vi "Chassis Info RTM.vi"(8 "error in (no error)":errorcluster, 11 "Node Ptr":u64 format="%.0x") -> (0 "error out":errorcluster)   [LabVIEW 2017, in "SLSC Switch System Explorer.lvlib"]
doc: "Demonstrates how to:\n- Discover SLSC devices\n- Reset SLSC devices\n- Rename SLSC devices\n- Add/remove SLSC chassis to/from the SLSC configuration file\n- Log in/out of an SLSC chassis, caching/deleting its login credentials\n- Update the firmware for an SLSC chassis\n- Open the web configuration page for an SLSC chassis"
uses:
  SLSC Switch System Explorer.lvlib
  SubVIs/ConfigurationStates.ctl
  <vilib>/NI Veristand/Custom Device API/Get Item Property (I32).vi
  <vilib>/nisyscfg/Close (System).vi
  <vilib>/SLSC/Initialize Session without Resources.vi
  <vilib>/SLSC/Initialize Session with Devices.vi
  <vilib>/SLSC/Close Session.vi
  <vilib>/Platform/browser.llb/Open URL in Default Browser (string).vi
  <vilib>/SLSC/SLSC.lvlib
  <resource>/objmgr/slsc.rc
  <vilib>/NI VeriStand/Custom Device API/Custom Device API.lvlib
  Scripting/VeriStand SLSC Scripting/VeriStand SLSC Scripting.lvlib
  <vilib>/nisyscfg/nisyscfg.lvlib
  <resource>/objmgr/nisysapi.rc
  <vilib>/Utility/SystemLogging/NI_SystemLogging.lvlib
panel:
  out "Name or IP":string
  out "Hostname":string
  in  "web config":bool
  in  "update firmware":bool
  out "device properties":string[][](table)
  in  "refresh":bool
  in  "logout":bool
  in  "login":bool
  in  "rename":bool
  in  "reset":bool
  in  "stop":bool
  in  "remove":bool
  in  "add":bool
  in  "devices":string(tree)="jasonSlsc-5"
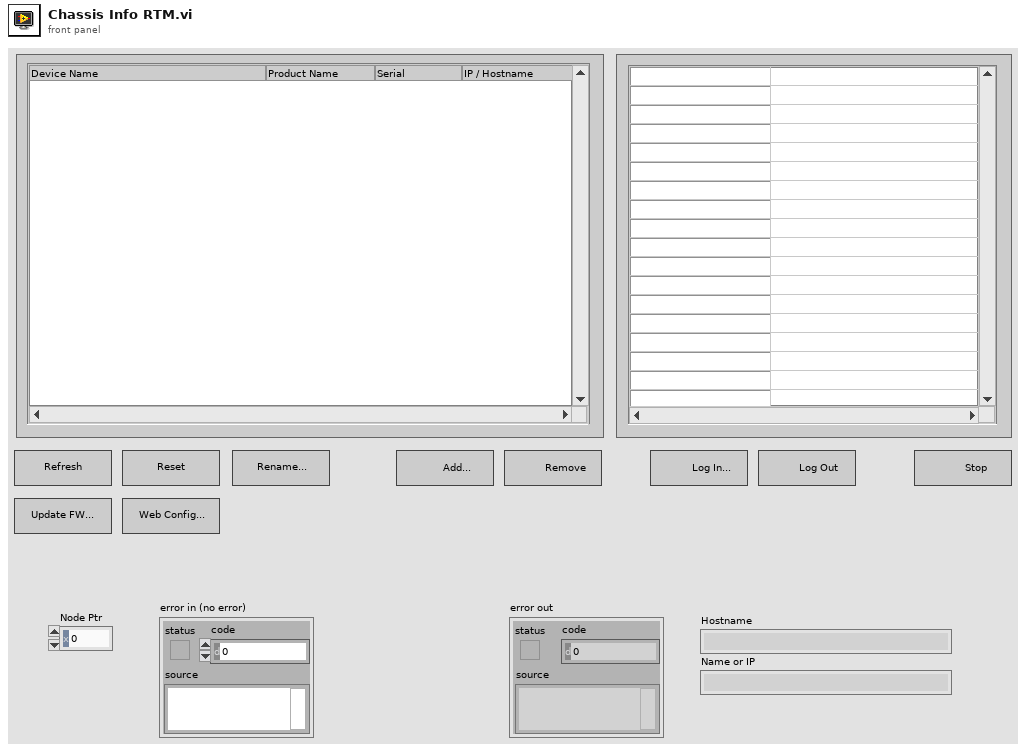
[diagram p1: front panel]
types:
  T1 = typedef "ConfigurationStates.ctl" = enum16{"Add", "Remove", "Rename", "Reset", "Login", "Logout", "Stop", "Refresh", "Update Firmware", "Web Config"}
  T2 = typedef "Custom Device API.lvlib/Custom Device Item Ref.ctl" = u64
  T3 = enum8{"Enabled", "Disabled", "Disabled and Grayed Out"}
  T4 = typedef "VeriStand SLSC Scripting.lvlib/SLSC Chassis ID.ctl" = cluster{"Name or IP":string, "ChassisIDType":i32, "chassisType":i32}
  T5 = enum32{"Invalid", "Standard", "Closed", "Hidden", "Minimized", "Maximized"}
  T6 = cluster{"hostname":string, "username":string, "password":string}
  T7 = cluster{"username":string, "password":string, "save credentials to disk":bool}
  T8 = cluster{"firmware path":path, "username":string, "password":string}
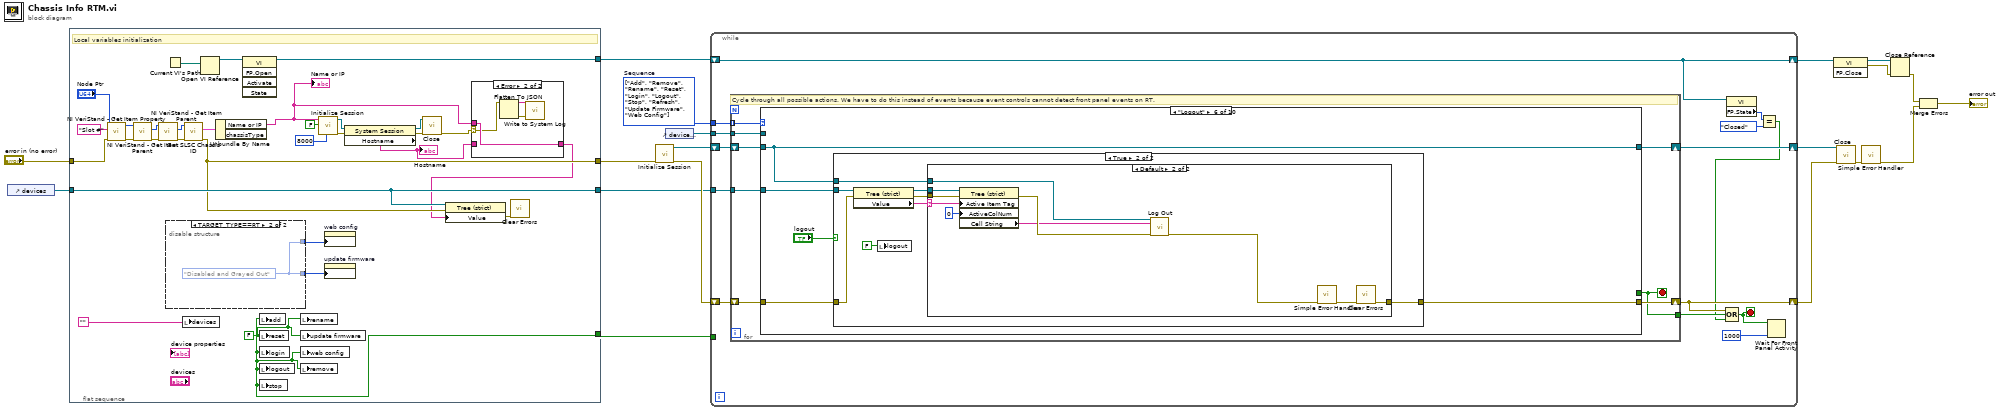
[diagram p0: block diagram]
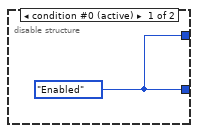
[diagram p3: hidden frame]
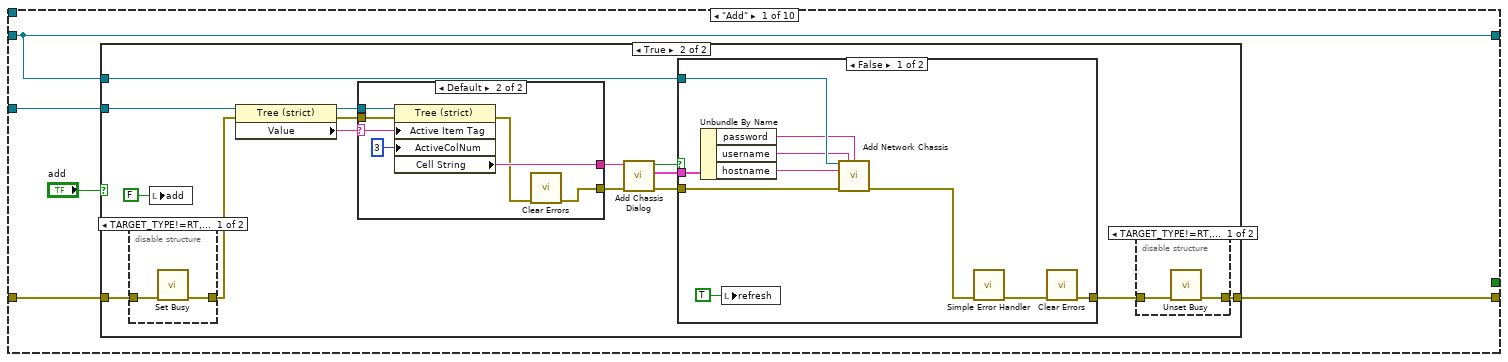
[diagram p4: hidden frame]
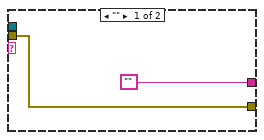
[diagram p6: hidden frame]
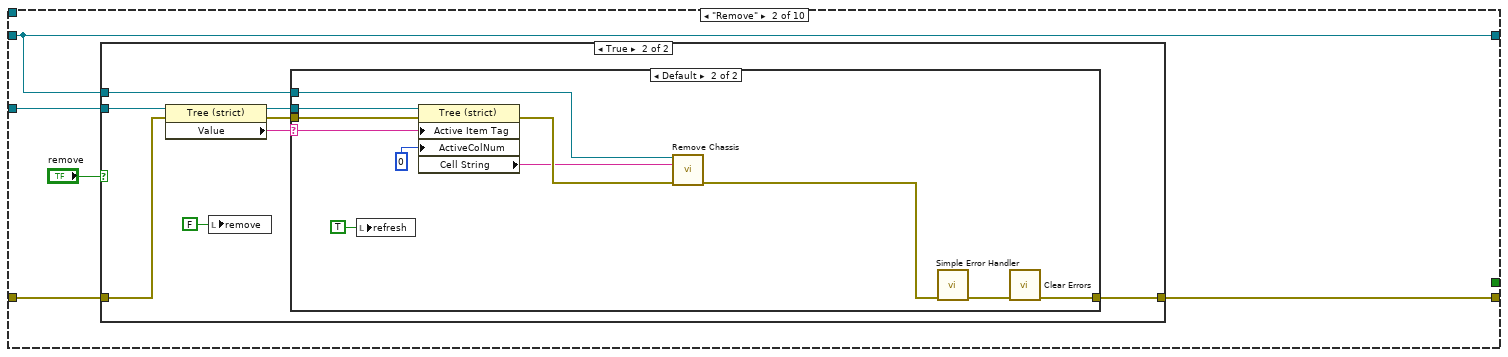
[diagram p10: hidden frame]
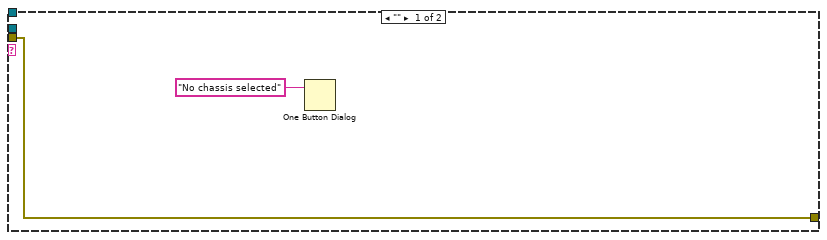
[diagram p12: hidden frame]
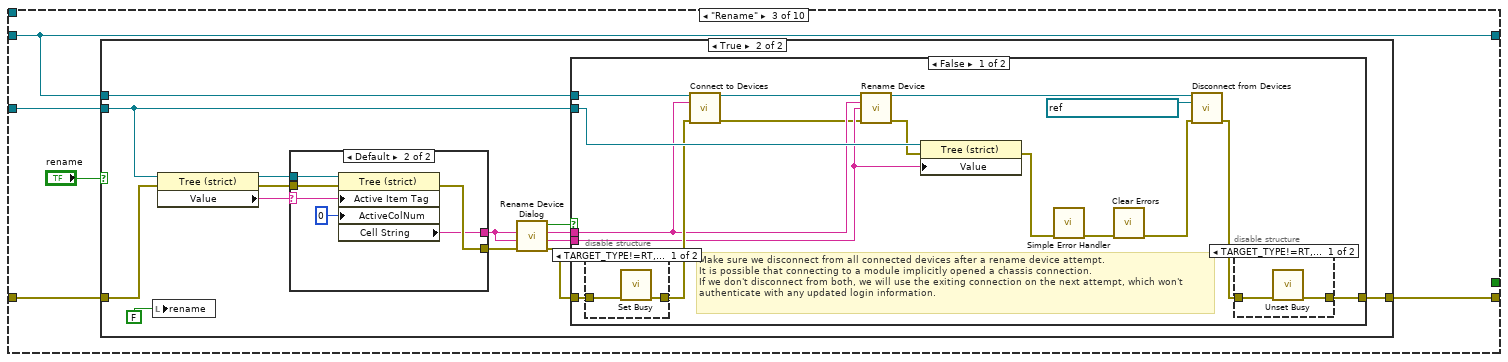
[diagram p13: hidden frame]
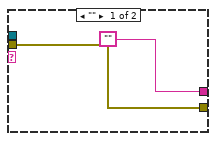
[diagram p15: hidden frame]
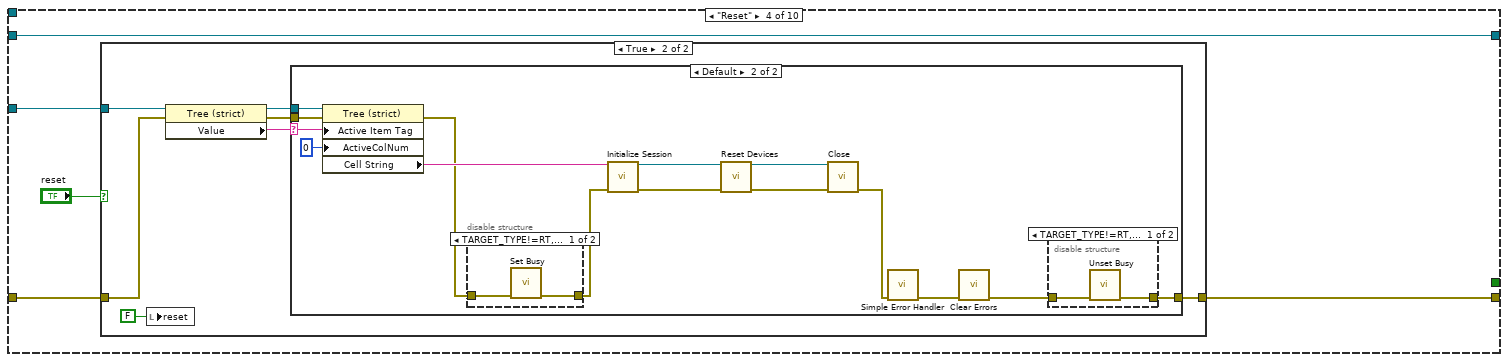
[diagram p19: hidden frame]
diagram:
  w15 = T1[] [enum."Add", enum."Remove", enum."Rename", enum."Reset", enum."Login", enum."Logout", enum."Stop", enum."Refresh", enum."Update Firmware", enum."Web Config"] items=["Add", "Remove", "Rename", "Reset", "Login", "Logout", "Stop", "Refresh", "Update Firmware", "Web Config"]  # Sequence
  n1 = control-ref of="devices"() -> (w6:refnum<vi>)
  n2 = flat-sequence {
    tunnel: [w49] -> w14
    tunnel: "error in (no error)" -> [w35]
    tunnel: [w24] -> w10
    tunnel: [w43] -> w9
    tunnel: [w34] -> w7
    tunnel: w6 -> [w34]
    frame #0 {
      w49 = FALSE
      # "Local variables initialization"
      n3 = call-poly <vilib>:"NI VeriStand - Get Item Property.vi"("error in (no error)"=w35, "Property Name"="Slot #", "Item Ref in"="Node Ptr") -> ("error out"=w39:errorcluster, "Item Ref out"=w38:T2)  [unwired: 5 in, 2 out]
      n4 = call <vilib>:"NI VeriStand - Get Item Parent.vi"("error in (no error)"=w39, "Item Ref in"=w38) -> ("error out"=w40:errorcluster, "Parent Ref"=w37:T2)  [unwired: 6 in, 2 out]
      n5 = call <vilib>:"NI VeriStand - Get Item Parent.vi"("error in (no error)"=w40, "Item Ref in"=w37) -> ("error out"=w41:errorcluster, "Parent Ref"=w32:T2)  [unwired: 6 in, 2 out]
      n6 = disable-structure shown="TARGET_TYPE==RT" {
        disable-tunnel: [w55 w56] -> w48
        disable-tunnel: [w55 w56] -> w46
        frame condition #0 (active) {
          w55 = T3."Enabled" ("Disabled")
        }
        frame condition #1 {
          w56 = T3."Disabled and Grayed Out" ("Disabled")
        }
      }
      n7 = Current VI's Path() -> (path=w45:path)
      n8 = local write "devices"("") -> ()
      n9 = call "Get SLSC Chassis ID.vi"("error in (no error)"=w41, "SLSC Chassis Ref in"=w32) -> ("error out"=w24:errorcluster, "SLSC Chassis ID"=w27:T4)  [unwired: 7 in, 1 out]
      n10 = Open VI Reference(vi path=w45) -> (vi reference=w44:refnum<vi>)  [unwired: 5 in, 1 out]
      n11 = Unbundle By Name(w27) -> ("Name or IP"=w20:string)  [unwired: 1 out]
      "Name or IP" <- w20
      n12 = invoke class="VI" method="FP.Open"(reference=w44) -> (reference out=w43:refnum<vi>)  [unwired: 4 in, 4 out]
      n13 = local write "add"(w49) -> ()
      n14 = local write "reset"(w49) -> ()
      n15 = local write "login"(w49) -> ()
      n16 = local write "logout"(w49) -> ()
      n17 = local write "stop"(w49) -> ()
      n18 = local write "rename"(w49) -> ()
      n19 = local write "update firmware"(w49) -> ()
      n20 = local write "web config"(w49) -> ()
      n21 = local write "remove"(w49) -> ()
      n22 = call <vilib>:"Initialize Session.vi"("Connect Timeout (4000 ms)"=u32 8000, "Force Property Refresh (T)"=FALSE, "Target (localhost)"=w20) -> ("error out"=w30:errorcluster, "Session out"=w31:refnum<k21>)  [unwired: 7 in]
      n23 = property on="web config" class="Bool (strict)"("DisabledEnum"=w46) -> ()  [unwired: 2 in, 2 out]
      n24 = property on="update firmware" class="Bool (strict)"("DisabledEnum"=w48) -> ()  [unwired: 2 in, 2 out]
      n25 = property class="System Session"(reference=w31, error in=w30) -> (reference out=w28:refnum<k21>, error out=w26:errorcluster, "Hostname"=w22:string)
      "Hostname" <- w22
      n26 = call-poly <vilib>:"Close.vi"("error in (no error)"=w26, "Session in"=w28) -> ("error out"=w23:errorcluster)  [unwired: 9 in]
      n27 = case shown="Error" w23 {
        selector: w23 -> [_ w51]
        tunnel: w22 -> [w50 _]
        tunnel: [w50 w54] -> w21
        tunnel: w20 -> [_ w54]
        frame No Error {
        }
        frame Error {
          n28 = Flatten To JSON(anything=w51) -> (JSON string=w52:string, 11:w53:errorcluster)  [unwired: 2 in]
          n29 = call <vilib>:"Write to System Log.vi"("error in (no error)"=w53, "message"=w52) -> ()  [unwired: 9 in, 1 out]
        }
      }
      n30 = property class="Tree (strict)"(reference=w34, error in=w24, "Value"=w21) -> (error out=w33:errorcluster)  [unwired: 1 out]
      n31 = call <vilib>:"Clear Errors.vi"("error in (no error)"=w33) -> ()  [unwired: 5 in, 2 out]
    }
  }
  n32 = call-poly <vilib>:"Initialize Session.vi"("error in (no error)"=w10) -> ("session out"=w16:refnum<k21>, "error out"=w19:errorcluster)  [unwired: 13 in]
  n33 = control-ref of="device properties"() -> (w12:refnum<vi>)
  n34 = while {
    shift-right: [w68] -> w18
    shift-left: w19 -> [w70]
    tunnel: w7 -> [w61]
    tunnel: w15 -> [w66]
    tunnel: w14 -> [_]
    shift-right: [w65] -> w13
    shift-left: w16 -> [w69]
    tunnel: w12 -> [w62]
    shift-right: [w60] -> w8
    shift-left: w9 -> [w60]
    stop <- w63 stop-if-true
    n35 = for {
      tunnel: [w73] -> w67
      tunnel: w61 -> [w75]
      shift-right: [w76] -> w68
      shift-left: w70 -> [w78]
      tunnel: w66 -> [w74] mode=indexing
      shift-right: [w72] -> w65
      shift-left: w69 -> [w77]
      tunnel: w62 -> [w71]
      stop <- w73 stop-if-true
      # "Cycle through all possible actions. We have to do this instead of events because event controls cannot detect front panel events on RT."
      n36 = case shown="\"Logout\"" w74 {
        tunnel: w78 -> [w82 w128 w156 w206 w243 w288 w313 w342 w413 w470]
        tunnel: w77 -> [w80 w126 w153 w204 w240 w285 w311 w334 w411 w472]
        tunnel: [w81 w127 w155 w205 w241 w286 w313 w319 w412 w469] -> w76
        tunnel: [_ _ _ _ _ _ "stop" _ _ _] -> w73
        tunnel: w75 -> [w79 w129 w157 w207 w242 w287 _ w336 w414 w473]
        tunnel: [w80 w126 w153 w204 w240 w285 w311 w339 w410 w471] -> w72
        tunnel: w71 -> [_ _ _ _ _ _ _ w337 _ _]
        frame "Add" {
          n37 = case shown="True" "add" {
            tunnel: w82 -> [w84 w98]
            tunnel: w80 -> [_ w97]
            tunnel: [w84 w96] -> w81
            tunnel: w79 -> [_ w85]
            frame False {
            }
            frame True {
              n38 = disable-structure shown="TARGET_TYPE!=RT, Default" {
                disable-tunnel: w98 -> [w113 w114]
                disable-tunnel: [w112 w114] -> w86
                frame condition #0 (active) {
                  n39 = call <vilib>:"Set Busy.vi"("error in (no error)"=w113) -> ("error out"=w112:errorcluster)  [unwired: 9 in, 1 out]
                }
                frame condition #1 {
                }
              }
              n40 = local write "add"(FALSE ("stop")) -> ()
              n41 = property class="Tree (strict)"(reference=w85, error in=w86) -> (reference out=w90:refnum<vi>, error out=w89:errorcluster, "Value"=w91:string)
              n42 = case shown="Default" w91 {
                selector: w91 -> [_ w104]
                tunnel: w89 -> [w101 w107]
                tunnel: w90 -> [_ w106]
                tunnel: [w101 w102] -> w87
                tunnel: ["" w105] -> w88
                frame "" {
                }
                frame Default {
                  n43 = property class="Tree (strict)"(reference=w106, error in=w107, "Active Item Tag"=w104, "ActiveColNum"=3 ("Active Cell:Active Column Number")) -> (error out=w103:errorcluster, "Cell String"=w105:string)  [unwired: 1 out]
                  n44 = call <vilib>:"Clear Errors.vi"("error in (no error)"=w103) -> ("error out"=w102:errorcluster)  [unwired: 5 in, 1 out]
                }
              }
              n45 = call "Add Chassis Dialog.vi"("error in (no error)"=w87, "hostname"=w88) -> ("error out"=w94:errorcluster, "Result"=w93:T6, "Cancelled?"=w95:bool)  [unwired: 7 in]
              n46 = case shown="False" w95 {
                tunnel: w97 -> [w124 _]
                tunnel: w93 -> [w123 _]
                tunnel: w94 -> [w121 w125]
                tunnel: [w118 w125] -> w99
                frame False {
                  n47 = Unbundle By Name(w123) -> ("password"=w116:string, "username"=w122:string, "hostname"=w115:string)
                  n48 = local write "refresh"(TRUE ("refresh")) -> ()
                  n49 = call <vilib>:"Add Network Chassis.vi"("session in"=w124, "username"=w122, "password"=w116, "chassis IP address/hostname"=w115, "error in (no error)"=w121) -> ("error out"=w120:errorcluster)  [unwired: 8 in, 2 out]
                  n50 = call <vilib>:"Simple Error Handler.vi"("error in (no error)"=w120) -> ("error out"=w119:errorcluster)  [unwired: 4 in, 4 out]
                  n51 = call <vilib>:"Clear Errors.vi"("error in (no error)"=w119) -> ("error out"=w118:errorcluster)  [unwired: 5 in, 1 out]
                }
                frame True {
                }
              }
              n52 = disable-structure shown="TARGET_TYPE!=RT, Default" {
                disable-tunnel: w99 -> [w110 w111]
                disable-tunnel: [w109 w111] -> w96
                frame condition #0 (active) {
                  n53 = call <vilib>:"Unset Busy.vi"("error in (no error)"=w110) -> ("error out"=w109:errorcluster)  [unwired: 10 in]
                }
                frame condition #1 {
                }
              }
            }
          }
        }
        frame "Remove" {
          n54 = case shown="True" "remove" {
            tunnel: w126 -> [_ w136]
            tunnel: w129 -> [_ w135]
            tunnel: w128 -> [w131 w134]
            tunnel: [w131 w133] -> w127
            frame False {
            }
            frame True {
              n55 = property class="Tree (strict)"(reference=w135, error in=w134) -> (reference out=w138:refnum<vi>, error out=w137:errorcluster, "Value"=w139:string)
              n56 = local write "remove"(FALSE ("stop")) -> ()
              n57 = case shown="Default" w139 {
                selector: w139 -> [_ w143]
                tunnel: w137 -> [w141 w151]
                tunnel: w138 -> [_ w150]
                tunnel: w136 -> [_ w149]
                tunnel: [w141 w147] -> w133
                frame "" {
                  n58 = One Button Dialog(message="No chassis selected") -> ()  [unwired: 1 in, 1 out]
                }
                frame Default {
                  n59 = local write "refresh"(TRUE ("refresh")) -> ()
                  n60 = property class="Tree (strict)"(reference=w150, error in=w151, "Active Item Tag"=w143, "ActiveColNum"=0 ("Active Cell:Active Column Number")) -> (error out=w148:errorcluster, "Cell String"=w144:string)  [unwired: 1 out]
                  n61 = call <vilib>:"Remove Chassis.vi"("session in"=w149, "chassis"=w144, "error in (no error)"=w148) -> ("error out"=w146:errorcluster)  [unwired: 11 in, 1 out]
                  n62 = call <vilib>:"Simple Error Handler.vi"("error in (no error)"=w146) -> ("error out"=w145:errorcluster)  [unwired: 4 in, 4 out]
                  n63 = call <vilib>:"Clear Errors.vi"("error in (no error)"=w145) -> ("error out"=w147:errorcluster)  [unwired: 5 in, 1 out]
                }
              }
            }
          }
        }
        frame "Rename" {
          n64 = case shown="True" "rename" {
            tunnel: w157 -> [_ w160]
            tunnel: w156 -> [w158 w162]
            tunnel: [w158 w164] -> w155
            tunnel: w153 -> [_ w159]
            frame False {
            }
            frame True {
              n65 = local write "rename"(FALSE ("stop")) -> ()
              n66 = property class="Tree (strict)"(reference=w160, error in=w162) -> (reference out=w171:refnum<vi>, error out=w170:errorcluster, "Value"=w172:string)
              n67 = case shown="Default" w172 {
                selector: w172 -> [_ w175]
                tunnel: w170 -> [w174 w179]
                tunnel: w171 -> [_ w178]
                tunnel: [w174 w177] -> w161
                tunnel: ["" w176] -> w165
                frame "" {
                }
                frame Default {
                  n68 = property class="Tree (strict)"(reference=w178, error in=w179, "Active Item Tag"=w175, "ActiveColNum"=0 ("Active Cell:Active Column Number")) -> (error out=w177:errorcluster, "Cell String"=w176:string)  [unwired: 1 out]
                }
              }
              n69 = call "Rename Device Dialog.vi"("error in (no error)"=w161, "new device name"=w165, "old device name"=w165) -> ("error out"=w163:errorcluster, "new device name out"=w167:string, "old device name out"=w168:string, "Cancelled?"=w169:bool)  [unwired: 5 in]
              n70 = case shown="False" w169 {
                tunnel: w168 -> [w190 _]
                tunnel: w167 -> [w189 _]
                tunnel: w163 -> [w194 w203]
                tunnel: [w195 w203] -> w164
                tunnel: w160 -> [w193 _]
                tunnel: w159 -> [w191 _]
                frame False {
                  # "Make sure we disconnect from all connected devices after a rename device attempt.\nIt is possible that connecting to a module implicitly opened a chassis connection.\nIf we don't disconnect from both, we will use the exiting connection on the next attempt, which won't authenticate with any updated login information."
                  n71 = disable-structure shown="TARGET_TYPE!=RT, Default" {
                    disable-tunnel: w194 -> [w197 w199]
                    disable-tunnel: [w198 w199] -> w192
                    frame condition #0 (active) {
                      n72 = call <vilib>:"Set Busy.vi"("error in (no error)"=w197) -> ("error out"=w198:errorcluster)  [unwired: 9 in, 1 out]
                    }
                    frame condition #1 {
                    }
                  }
                  n73 = call <vilib>:"Connect to Devices.vi"("session in"=w191, "devices"=w190, "error in (no error)"=w192) -> ("session out"=w187:refnum<k21>, "error out"=w186:errorcluster)  [unwired: 11 in]
                  n74 = call <vilib>:"Rename Device.vi"("session in"=w187, "device"=w190, "new device name"=w189, "error in (no error)"=w186) -> ("session out"=w183:refnum<k21>, "error out"=w185:errorcluster)  [unwired: 10 in]
                  n75 = property class="Tree (strict)"(reference=w193, error in=w185, "Value"=w189) -> (error out=w188:errorcluster)  [unwired: 1 out]
                  n76 = call <vilib>:"Simple Error Handler.vi"("error in (no error)"=w188) -> ("error out"=w196:errorcluster)  [unwired: 4 in, 4 out]
                  n77 = call <vilib>:"Clear Errors.vi"("error in (no error)"=w196) -> ("error out"=w181:errorcluster)  [unwired: 5 in, 1 out]
                  n78 = call <vilib>:"Disconnect from Devices.vi"("session in"=w183, "devices"=refnum<k21> "$ConnectedDevices", "error in (no error)"=w181) -> ("error out"=w184:errorcluster)  [unwired: 11 in, 1 out]
                  n79 = disable-structure shown="TARGET_TYPE!=RT, Default" {
                    disable-tunnel: w184 -> [w201 w202]
                    disable-tunnel: [w200 w202] -> w195
                    frame condition #0 (active) {
                      n80 = call <vilib>:"Unset Busy.vi"("error in (no error)"=w201) -> ("error out"=w200:errorcluster)  [unwired: 10 in]
                    }
                    frame condition #1 {
                    }
                  }
                }
                frame True {
                }
              }
            }
          }
        }
        frame "Reset" {
          n81 = case shown="True" "reset" {
            tunnel: w207 -> [_ w214]
            tunnel: w206 -> [w209 w213]
            tunnel: [w209 w210] -> w205
            frame False {
            }
            frame True {
              n82 = local write "reset"(FALSE ("stop")) -> ()
              n83 = property class="Tree (strict)"(reference=w214, error in=w213) -> (reference out=w215:refnum<vi>, error out=w211:errorcluster, "Value"=w216:string)
              n84 = case shown="Default" w216 {
                selector: w216 -> [_ w229]
                tunnel: w211 -> [w218 w232]
                tunnel: w215 -> [_ w231]
                tunnel: [w218 w219] -> w210
                frame "" {
                  n85 = One Button Dialog(message="No device selected") -> ()  [unwired: 1 in, 1 out]
                }
                frame Default {
                  n86 = property class="Tree (strict)"(reference=w231, error in=w232, "Active Item Tag"=w229, "ActiveColNum"=0 ("Active Cell:Active Column Number")) -> (error out=w222:errorcluster, "Cell String"=w226:string)  [unwired: 1 out]
                  n87 = disable-structure shown="TARGET_TYPE!=RT, Default" {
                    disable-tunnel: w222 -> [w238 w239]
                    disable-tunnel: [w237 w239] -> w221
                    frame condition #0 (active) {
                      n88 = call <vilib>:"Set Busy.vi"("error in (no error)"=w238) -> ("error out"=w237:errorcluster)  [unwired: 9 in, 1 out]
                    }
                    frame condition #1 {
                    }
                  }
                  n89 = call-poly <vilib>:"Initialize Session.vi"("devices"=w226, "error in (no error)"=w221) -> ("session out"=w228:refnum<k21>, "error out"=w227:errorcluster)  [unwired: 12 in]
                  n90 = call <vilib>:"Reset Devices.vi"("session in"=w228, "error in (no error)"=w227) -> ("session out"=w223:refnum<k21>, "error out"=w225:errorcluster)  [unwired: 12 in]
                  n91 = call-poly <vilib>:"Close.vi"("session in"=w223, "error in (no error)"=w225) -> ("error out"=w224:errorcluster)  [unwired: 13 in]
                  n92 = call <vilib>:"Simple Error Handler.vi"("error in (no error)"=w224) -> ("error out"=w230:errorcluster)  [unwired: 4 in, 4 out]
                  n93 = call <vilib>:"Clear Errors.vi"("error in (no error)"=w230) -> ("error out"=w220:errorcluster)  [unwired: 5 in, 1 out]
                  n94 = disable-structure shown="TARGET_TYPE!=RT, Default" {
                    disable-tunnel: w220 -> [w235 w236]
                    disable-tunnel: [w234 w236] -> w219
                    frame condition #0 (active) {
                      n95 = call <vilib>:"Unset Busy.vi"("error in (no error)"=w235) -> ("error out"=w234:errorcluster)  [unwired: 10 in]
                    }
                    frame condition #1 {
                    }
                  }
                }
              }
            }
          }
        }
        frame "Login" {
          n96 = case shown="True" "login" {
            tunnel: w240 -> [_ w250]
            tunnel: w243 -> [w245 w249]
            tunnel: w242 -> [_ w248]
            tunnel: [w245 w247] -> w241
            frame False {
            }
            frame True {
              n97 = local write "login"(FALSE ("stop")) -> ()
              n98 = property class="Tree (strict)"(reference=w248, error in=w249) -> (reference out=w252:refnum<vi>, error out=w251:errorcluster, "Value"=w253:string)
              n99 = case shown="Default" w253 {
                selector: w253 -> [_ w264]
                tunnel: w251 -> [w254 w266]
                tunnel: w252 -> [_ w265]
                tunnel: [w254 w259] -> w247
                tunnel: w250 -> [_ w262]
                frame "" {
                }
                frame Default {
                  n100 = property class="Tree (strict)"(reference=w265, error in=w266, "Active Item Tag"=w264, "ActiveColNum"=0 ("Active Cell:Active Column Number")) -> (error out=w261:errorcluster, "Cell String"=w263:string)  [unwired: 1 out]
                  n101 = disable-structure shown="TARGET_TYPE!=RT, Default" {
                    disable-tunnel: w261 -> [w272 w273]
                    disable-tunnel: [w271 w273] -> w256
                    frame condition #0 (active) {
                      n102 = call <vilib>:"Set Busy.vi"("error in (no error)"=w272) -> ("error out"=w271:errorcluster)  [unwired: 9 in, 1 out]
                    }
                    frame condition #1 {
                    }
                  }
                  n103 = call "Log In Dialog.vi"("error in (no error)"=w256) -> ("error out"=w255:errorcluster, "Result"=w257:T7, "Cancelled?"=w258:bool)  [unwired: 8 in]
                  n104 = case shown="False" w258 {
                    tunnel: w257 -> [w283 _]
                    tunnel: w255 -> [w282 w284]
                    tunnel: [w279 w284] -> w260
                    tunnel: w263 -> [w278 _]
                    tunnel: w262 -> [w277 _]
                    frame False {
                      n105 = Unbundle By Name(w283) -> ("password"=w274:string, "username"=w276:string, "save credentials to disk"=w275:bool)
                      n106 = call <vilib>:"Log In.vi"("session in"=w277, "username"=w276, "password"=w274, "chassis"=w278, "error in (no error)"=w282, "save credentials to disk? (F)"=w275) -> ("error out"=w281:errorcluster)  [unwired: 8 in, 1 out]
                      n107 = call <vilib>:"Simple Error Handler.vi"("error in (no error)"=w281) -> ("error out"=w280:errorcluster)  [unwired: 4 in, 4 out]
                      n108 = call <vilib>:"Clear Errors.vi"("error in (no error)"=w280) -> ("error out"=w279:errorcluster)  [unwired: 5 in, 1 out]
                    }
                    frame True {
                    }
                  }
                  n109 = disable-structure shown="TARGET_TYPE!=RT, Default" {
                    disable-tunnel: w260 -> [w269 w270]
                    disable-tunnel: [w268 w270] -> w259
                    frame condition #0 (active) {
                      n110 = call <vilib>:"Unset Busy.vi"("error in (no error)"=w269) -> ("error out"=w268:errorcluster)  [unwired: 10 in]
                    }
                    frame condition #1 {
                    }
                  }
                }
              }
            }
          }
        }
        frame "Logout" {
          n111 = case shown="True" "logout" {
            tunnel: w285 -> [_ w295]
            tunnel: w288 -> [w290 w294]
            tunnel: w287 -> [_ w293]
            tunnel: [w290 w292] -> w286
            frame False {
            }
            frame True {
              n112 = property class="Tree (strict)"(reference=w293, error in=w294) -> (reference out=w297:refnum<vi>, error out=w296:errorcluster, "Value"=w298:string)
              n113 = local write "logout"(FALSE ("stop")) -> ()
              n114 = case shown="Default" w298 {
                selector: w298 -> [_ w301]
                tunnel: w296 -> [w300 w309]
                tunnel: w297 -> [_ w308]
                tunnel: w295 -> [_ w307]
                tunnel: [w300 w305] -> w292
                frame "" {
                  n115 = One Button Dialog(message="No chassis selected") -> ()  [unwired: 1 in, 1 out]
                }
                frame Default {
                  n116 = property class="Tree (strict)"(reference=w308, error in=w309, "Active Item Tag"=w301, "ActiveColNum"=0 ("Active Cell:Active Column Number")) -> (error out=w306:errorcluster, "Cell String"=w302:string)  [unwired: 1 out]
                  n117 = call <vilib>:"Log Out.vi"("session in"=w307, "chassis"=w302, "error in (no error)"=w306) -> ("error out"=w304:errorcluster)  [unwired: 11 in, 1 out]
                  n118 = call <vilib>:"Simple Error Handler.vi"("error in (no error)"=w304) -> ("error out"=w303:errorcluster)  [unwired: 4 in, 4 out]
                  n119 = call <vilib>:"Clear Errors.vi"("error in (no error)"=w303) -> ("error out"=w305:errorcluster)  [unwired: 5 in, 1 out]
                }
              }
            }
          }
        }
        frame "Stop" {
          n120 = case shown="True" "stop" {
            frame False {
            }
            frame True {
              n121 = local write "stop"(FALSE ("stop")) -> ()
            }
          }
        }
        frame "Refresh" {
          n122 = disable-structure shown="TARGET_TYPE!=RT, Default" {
            disable-tunnel: w342 -> [w404 w408]
            disable-tunnel: [w403 w408] -> w316
            disable-tunnel: [w402 _] -> w343
            frame condition #0 (active) {
              n123 = property class="VI"(error in=w404) -> (error out=w406:errorcluster, "Panel"=w407:refnum<vi>)  [unwired: 1 in, 1 out]
              n124 = property class="Pnl"(reference=w407, error in=w406, "DeferPanUpdts"=TRUE ("Defer Panel Updates")) -> (reference out=w402:refnum<vi>, error out=w403:errorcluster)
            }
            frame condition #1 {
            }
          }
          n125 = case shown="True" "refresh" {
            tunnel: [w389 w391] -> w315
            tunnel: w316 -> [w389 w390]
            frame False {
            }
            frame True {
              n126 = local write "refresh"(FALSE ("refresh")) -> ()
              n127 = invoke on="devices" class="Tree (strict)" method="Edit Tree Items.Delete"("tag"="", "Delete Children"=TRUE ("refresh")) -> (error out=w392:errorcluster)  [unwired: 3 in, 4 out]
              n128 = Merge Errors(w392, w390) -> (w391:errorcluster)
            }
          }
          n129 = property class="SLSC Session"(reference=w334, error in=w315) -> (reference out=w333:refnum<k21>, error out=w332:errorcluster, "Sys.ConfigChangeCount"=w329:u64)
          n130 = feedback #1(u64 0 ("Sys.ConfigChangeCount")) -> (w330:u64)
          n131 = feedback-in #1(w329) -> ()
          n132 = Not Equal?(x=w329, y=w330) -> (x != y?=w327:bool)
          n133 = Or(x=w327, y="refresh") -> (x .or. y?=w328:bool)
          n134 = case shown="True" w328 {
            tunnel: [w352 w360] -> w341
            tunnel: [w354 w359] -> w340
            tunnel: w336 -> [w353 w358]
            tunnel: [w353 w357] -> w335
            tunnel: w333 -> [w354 w356]
            tunnel: w332 -> [w352 w355]
            frame False {
            }
            frame True {
              n135 = call "Update Config Tree.vi"("error in (no error)"=w355, "devices"=w358, "session in"=w356) -> ("error out"=w360:errorcluster, "devices out"=w357:refnum<vi>, "session out"=w359:refnum<k21>)  [unwired: 6 in]
            }
          }
          n136 = property class="Tree (strict)"(reference=w335, error in=w341) -> (reference out=w323:refnum<vi>, error out=w322:errorcluster, "Value"=w318:string, "All Tags"=w325:string[])
          n137 = Search 1D Array(1D array=w325, element=w318) -> (index of element=w324:i32)  [unwired: 1 in]
          n138 = case shown="-1" w324 {
            tunnel: w323 -> [w345 w350]
            tunnel: w322 -> [w346 w351]
            tunnel: [w345 w349] -> w321
            tunnel: [w346 w348] -> w320
            tunnel: w318 -> [w344 _]
            tunnel: [w344 w347] -> w317
            frame Default {
              # "Tag is valid"
            }
            frame -1 {
              w347 = ""
              # "Tag is no longer valid. Clear control value to avoid accessing invalid tree items."
              n139 = property class="Tree (strict)"(reference=w350, error in=w351, "Value"=w347) -> (reference out=w349:refnum<vi>, error out=w348:errorcluster)
            }
          }
          n140 = case shown="Default" w317 {
            selector: w317 -> [_ w380]
            tunnel: w340 -> [w364 w379]
            tunnel: [w364 w373] -> w339
            tunnel: w320 -> [w365 w375]
            tunnel: w321 -> [_ w378]
            tunnel: [w366 w374] -> w338
            tunnel: "refresh" -> [_ w377]
            tunnel: w337 -> [w361 w376]
            frame "" {
              n141 = property class="Tbl (strict)"(reference=w361, error in=w365, "Row Headers[]"=string[] [] ("Row Header Strings[]"), "Value"=string[][] []) -> (error out=w366:errorcluster)  [unwired: 1 out]
            }
            frame Default {
              n142 = property class="Tree (strict)"(reference=w378, error in=w375, "Active Item Tag"=w380, "ActiveColNum"=0 ("Active Cell:Active Column Number")) -> (error out=w371:errorcluster, "Cell String"=w368:string)  [unwired: 1 out]
              n143 = feedback #2() -> (w367:string)  [unwired: 1 in]
              n144 = feedback-in #2(w368) -> ()
              n145 = Not Equal?(x=w368, y=w367) -> (x != y?=w370:bool)
              n146 = Or(x=w370, y=w377) -> (x .or. y?=w369:bool)
              n147 = case shown="True" w369 {
                tunnel: w368 -> [_ w388]
                tunnel: w371 -> [w381 w387]
                tunnel: w379 -> [w382 w386]
                tunnel: [w382 w385] -> w373
                tunnel: [w381 w384] -> w374
                tunnel: w376 -> [_ w383]
                frame False {
                }
                frame True {
                  n148 = call "Update Device Properties Table.vi"("session in"=w386, "device"=w388, "device properties"=w383, "error in (no error)"=w387) -> ("session out"=w385:refnum<k21>, "error out"=w384:errorcluster)  [unwired: 10 in]
                }
              }
            }
          }
          n149 = disable-structure shown="TARGET_TYPE!=RT, Default" {
            disable-tunnel: w343 -> [w400 _]
            disable-tunnel: w338 -> [w397 w401]
            disable-tunnel: [w396 w401] -> w319
            frame condition #0 (active) {
              n150 = property class="Pnl"(reference=w400, "DeferPanUpdts"=FALSE ("Defer Panel Updates")) -> (error out=w398:errorcluster)  [unwired: 1 in, 1 out]
              n151 = Merge Errors(w397, w398) -> (w396:errorcluster)
            }
            frame condition #1 {
            }
          }
        }
        frame "Update Firmware" {
          n152 = case shown="True" "update firmware" {
            tunnel: w414 -> [_ w422]
            tunnel: w413 -> [w416 w420]
            tunnel: [w416 w419] -> w412
            tunnel: w411 -> [w415 w418]
            tunnel: [w415 w417] -> w410
            frame False {
            }
            frame True {
              n153 = local write "update firmware"(FALSE ("update firmware")) -> ()
              n154 = disable-structure shown="Default" {
                disable-tunnel: w422 -> [w429 _]
                disable-tunnel: w420 -> [w428 w466]
                disable-tunnel: [w425 w466] -> w419
                disable-tunnel: w418 -> [w424 w467]
                disable-tunnel: [w423 w467] -> w417
                frame condition #0 (active) {
                  n155 = disable-structure shown="TARGET_TYPE!=RT, Default" {
                    disable-tunnel: w428 -> [w437 w438]
                    disable-tunnel: [w436 w438] -> w427
                    frame condition #0 (active) {
                      n156 = call <vilib>:"Set Busy.vi"("error in (no error)"=w437) -> ("error out"=w436:errorcluster)  [unwired: 9 in, 1 out]
                    }
                    frame condition #1 {
                    }
                  }
                  n157 = property class="Tree (strict)"(reference=w429, error in=w427) -> (reference out=w431:refnum<vi>, error out=w430:errorcluster, "Value"=w432:string)
                  n158 = case shown="Default" w432 {
                    selector: w432 -> [_ w449]
                    tunnel: w430 -> [w440 w451]
                    tunnel: w431 -> [_ w450]
                    tunnel: [w440 w443] -> w426
                    tunnel: w424 -> [w439 w442]
                    tunnel: [w439 w441] -> w423
                    frame "" {
                    }
                    frame Default {
                      n159 = property class="Tree (strict)"(reference=w450, error in=w451, "Active Item Tag"=w449, "ActiveColNum"=0 ("Active Cell:Active Column Number")) -> (error out=w448:errorcluster, "Cell String"=w445:string)  [unwired: 1 out]
                      n160 = call "Update Firmware Dialog.vi"("error in (no error)"=w448) -> ("error out"=w444:errorcluster, "Result"=w446:T8, "Cancelled?"=w447:bool)  [unwired: 8 in]
                      n161 = case shown="False" w447 {
                        tunnel: w446 -> [w463 _]
                        tunnel: w445 -> [w453 _]
                        tunnel: w444 -> [w456 w465]
                        tunnel: [w461 w465] -> w443
                        tunnel: w442 -> [w460 w464]
                        tunnel: [w454 w464] -> w441
                        frame False {
                          n162 = Unbundle By Name(w463) -> ("password"=w458:string, "username"=w459:string, "firmware path"=w457:path)
                          n163 = call <vilib>:"Update Chassis Firmware.vi"("session in"=w460, "username"=w459, "password"=w458, "chassis"=w453, "firmware path"=w457, "error in (no error)"=w456) -> ("session out"=w454:refnum<k21>, "error out"=w455:errorcluster)  [unwired: 8 in]
                          n164 = call <vilib>:"Simple Error Handler.vi"("error in (no error)"=w455) -> ("error out"=w462:errorcluster)  [unwired: 4 in, 4 out]
                          n165 = call <vilib>:"Clear Errors.vi"("error in (no error)"=w462) -> ("error out"=w461:errorcluster)  [unwired: 5 in, 1 out]
                        }
                        frame True {
                        }
                      }
                    }
                  }
                  n166 = disable-structure shown="TARGET_TYPE!=RT, Default" {
                    disable-tunnel: w426 -> [w434 w435]
                    disable-tunnel: [w433 w435] -> w425
                    frame condition #0 (active) {
                      n167 = call <vilib>:"Unset Busy.vi"("error in (no error)"=w434) -> ("error out"=w433:errorcluster)  [unwired: 10 in]
                    }
                    frame condition #1 {
                    }
                  }
                }
                frame condition #1 {
                  n168 = One Button Dialog(message="Firmware update is not supported on this platform.") -> ()  [unwired: 1 in, 1 out]
                }
              }
            }
          }
        }
        frame "Web Config" {
          n169 = case shown="True" "web config" {
            tunnel: w472 -> [w475 w480]
            tunnel: w473 -> [_ w481]
            tunnel: [w475 w479] -> w471
            tunnel: w470 -> [w476 w478]
            tunnel: [w476 w477] -> w469
            frame False {
            }
            frame True {
              n170 = local write "web config"(FALSE ("web config")) -> ()
              n171 = disable-structure shown="Default" {
                disable-tunnel: w481 -> [w490 _]
                disable-tunnel: w480 -> [w487 _]
                disable-tunnel: [w486 _] -> w479
                disable-tunnel: w478 -> [w485 _]
                disable-tunnel: [w484 _] -> w477
                frame condition #0 (active) {
                  n172 = property class="Tree (strict)"(reference=w490, error in=w485) -> (reference out=w483:refnum<vi>, error out=w488:errorcluster, "Value"=w489:string)
                  n173 = case shown="Default" w489 {
                    selector: w489 -> [_ w496]
                    tunnel: w488 -> [w491 w506]
                    tunnel: w487 -> [w492 w504]
                    tunnel: [w492 w503] -> w486
                    tunnel: [w491 w493] -> w484
                    tunnel: w483 -> [_ w497]
                    frame "" {
                    }
                    frame Default {
                      n174 = property class="Tree (strict)"(reference=w497, error in=w506, "Active Item Tag"=w496, "ActiveColNum"=0 ("Active Cell:Active Column Number")) -> (error out=w502:errorcluster, "Cell String"=w505:string)  [unwired: 1 out]
                      n175 = call <vilib>:"Get Chassis IP or Hostname.vi"("session in"=w504, "chassis"=w505, "error in (no error)"=w502) -> ("session out"=w503:refnum<k21>, "chassis IP address/hostname"=w500:string, "error out"=w498:errorcluster)  [unwired: 10 in]
                      n176 = Concatenate Strings("http://", w500) -> (w499:string)
                      n177 = call-poly <vilib>:"Open URL in Default Browser.vi"("error in (no error)"=w498, "URL"=w499) -> ("error out"=w494:errorcluster)  [unwired: 4 in, 1 out]
                      n178 = call <vilib>:"Simple Error Handler.vi"("error in (no error)"=w494) -> ("error out"=w495:errorcluster)  [unwired: 4 in, 4 out]
                      n179 = call <vilib>:"Clear Errors.vi"("error in (no error)"=w495) -> ("error out"=w493:errorcluster)  [unwired: 5 in, 1 out]
                    }
                  }
                }
                frame condition #1 {
                  n180 = One Button Dialog(message="Opening a web browser is not supported on this platform.") -> ()  [unwired: 1 in, 1 out]
                }
              }
            }
          }
        }
      }
    }
    n181 = property class="VI"(reference=w60) -> ("FP.State"=w59:T5)  [unwired: 1 in, 2 out]
    n182 = Equal?(x=w59, y=T5."Closed" ("Front Panel Window:State")) -> (x = y?=w57:bool)
    n183 = Compound Arithmetic op=OR(w68, w67, w57) -> (w63:bool)
    n184 = Wait For Front Panel Activity(1:1000 ("timeout ms (-1 never timeout)"), 3:w63) -> ()  [unwired: 1 in, 1 out]
  }
  n185 = invoke class="VI" method="FP.Close"(reference=w8) -> (reference out=w5:refnum<vi>, error out=w4:errorcluster)  [unwired: 2 in, 1 out]
  n186 = call-poly <vilib>:"Close.vi"("session in"=w13, "error in (no error)"=w18) -> ("error out"=w17:errorcluster)  [unwired: 13 in]
  n187 = call <vilib>:"Simple Error Handler.vi"("error in (no error)"=w17) -> ("error out"=w2:errorcluster)  [unwired: 4 in, 4 out]
  n188 = Close Reference(reference=w5, error in (no error)=w4) -> (error out=w3:errorcluster)
  n189 = Merge Errors(w3, w2) -> (→"error out":errorcluster)
